vi "update_jv_log.vi"(0 "File path for master log":path, 1 "Cell details cluster":T1={"Cell Position"=16, "Cell Label"="", "Pixel to measure"=0, "Area (cm^2)"=0.126, "Variable"="", "Variable value"="", "Scan settings in queue"=0, "Light or dark"="", "Measurement type"=""} {"Pixel to measure" items=["All", "1", "2", "3", "4", "5", "6", "7", "8"]}, 5 "j-v metrics":string[](array[string]), 11 "scan number":string) -> (4 "File path for master log":path)   [LabVIEW 2016]
uses:
  <vilib>/Utility/file.llb/Write Delimited Spreadsheet (string).vi
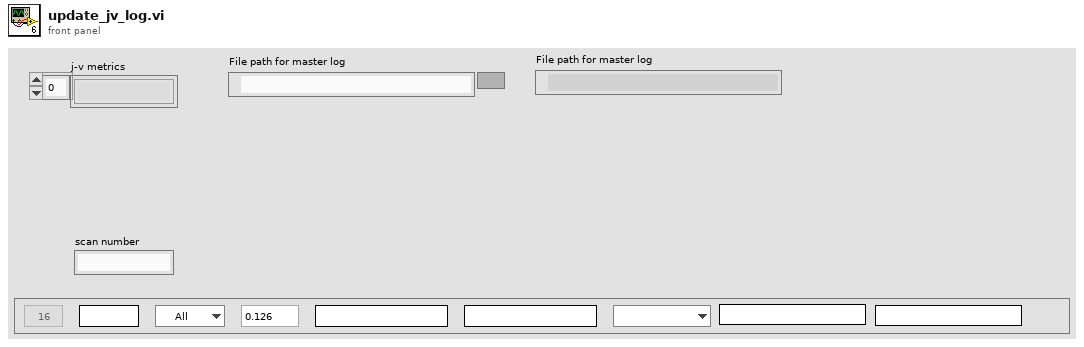
[diagram p1: front panel]
types:
  T1 = cluster{"Cell Position":i32, "Cell Label":string, "Pixel to measure":u16, "Area (cm^2)":dbl, "Variable":string, "Variable value":string, "Scan settings in queue":u16, "Light or dark":string, "Measurement type":string}
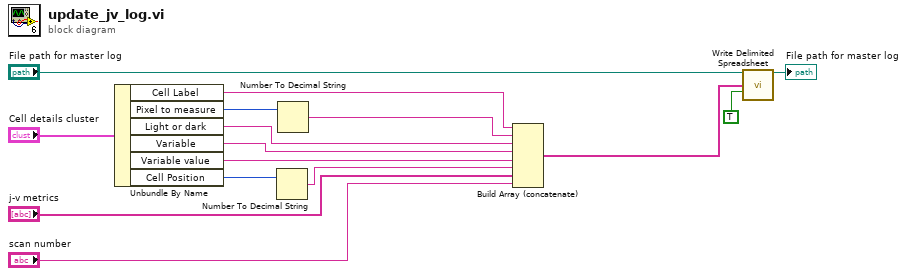
[diagram p0: block diagram]
diagram:
  n1 = Unbundle By Name("Cell details cluster") -> ("Cell Label"=w12:string, "Pixel to measure"=w11:u16, "Light or dark"=w9:string, "Variable"=w8:string, "Variable value"=w7:string, "Cell Position"=w6:i32)
  n2 = Number To Decimal String(number=w6) -> (decimal integer string=w5:string)  [unwired: 1 in]
  n3 = Number To Decimal String(number=w11) -> (decimal integer string=w10:string)  [unwired: 1 in]
  n4 = Build Array (concatenate)(w12, w10, w9, w8, w7, w5, "j-v metrics", "scan number") -> (w14:string[])
  n5 = call-poly <vilib>:"Write Delimited Spreadsheet.vi"("file path (dialog if empty)"="File path for master log", "1D data"=w14, "append to file? (new file:F)"=TRUE) -> ("new file path (Not A Path if cancelled)"=→"File path for master log":path)  [unwired: 11 in, 1 out]
